vi "Translator.vi"(0 "Input":variant, 11 "error in (no error)":errorcluster) -> (4 "Output":variant, 15 "error out":errorcluster)   [LabVIEW 2014, in "Arduino Extra Functions.lvlib"]
doc: "An example of how to create the Translator to convert the LabVIEW VIs to Arduino C code."
uses:
  <vilib>/Aledyne-TSXperts/Arduino Compatible Compiler for LabVIEW/addons/Arduino Extra Functions/Arduino Extra Functions.lvlib
panel:
  out "Outputs":string[](array[string])
  out "Inputs":string[](array[string])
  out "Output Datatypes":string[](array[string])
  out "Input Datatypes":string[](array[string])
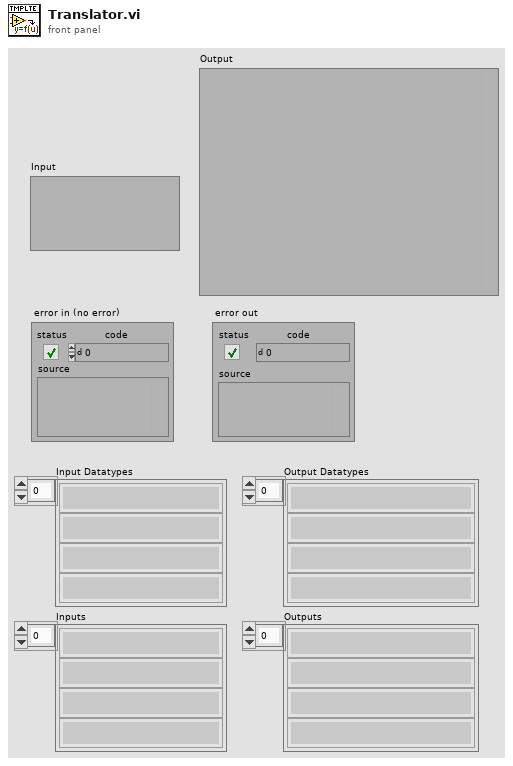
[diagram p1: front panel]
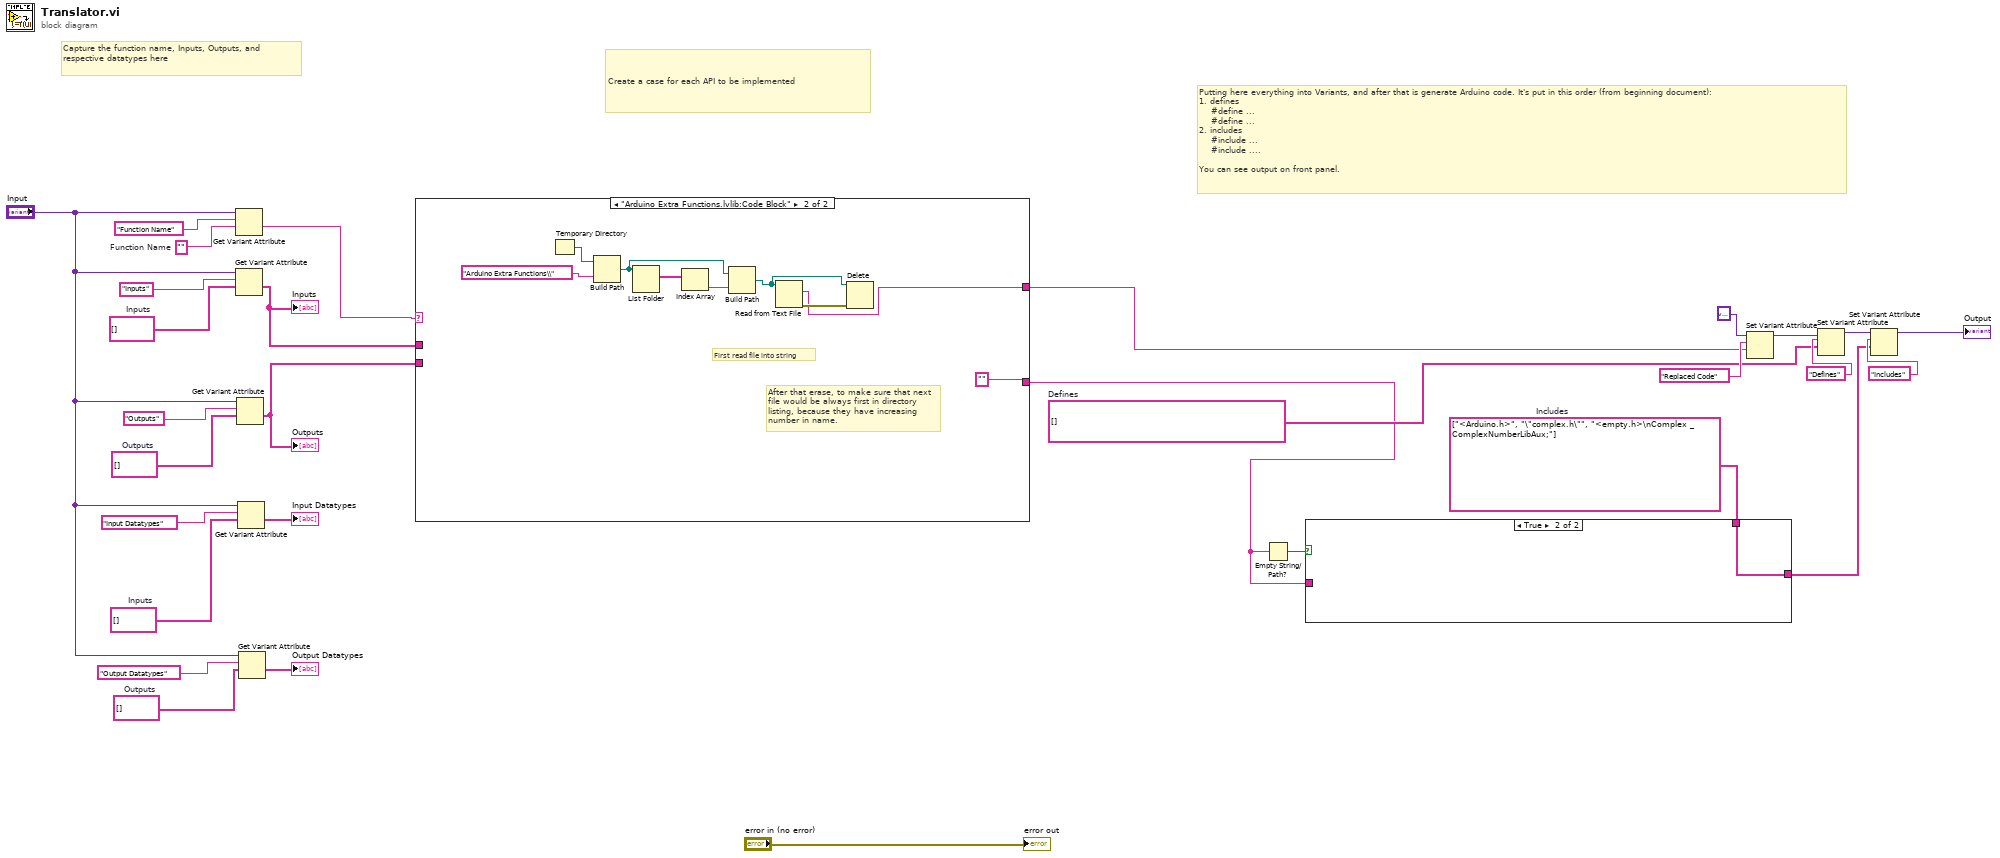
[diagram p0: block diagram]
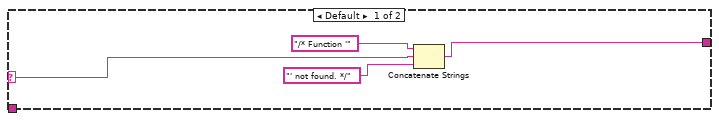
[diagram p2: hidden frame]
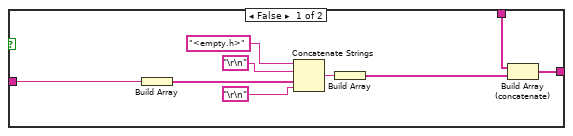
[diagram p3: hidden frame]
diagram:
  w8 = string[] []  # Defines
  w19 = string[] []  # Outputs
  w20 = string[] []  # Inputs
  w6 = string[] ["<Arduino.h>", "\"complex.h\"", "<empty.h>\nComplex _ComplexNumberLibAux;"]  # Includes
  w26 = string[] []  # Outputs
  w27 = string[] []  # Inputs
  w28 = ""  # Function Name
  # "Capture the function name, Inputs, Outputs, and respective datatypes here"
  # "Putting here everything into Variants, and after that is generate Arduino code. It's put in this order (from beginning document):\n1. defines\n    #define ...\n    #define ...\n2. includes\n    #include ...\n    #include ....\n\nYou can see output on front panel."
  # "Create a case for each API to be implemented"
  n1 = Get Variant Attribute(Variant="Input", name="Function Name", default value (empty Variant)=w28) -> (value=w5:string)  [unwired: 1 in, 3 out]
  n2 = Get Variant Attribute(Variant="Input", name="Inputs", default value (empty Variant)=w27) -> (value=w4:string[])  [unwired: 1 in, 3 out]
  "Inputs" <- w4
  n3 = Get Variant Attribute(Variant="Input", name="Outputs", default value (empty Variant)=w26) -> (value=w3:string[])  [unwired: 1 in, 3 out]
  "Outputs" <- w3
  n4 = Get Variant Attribute(Variant="Input", name="Input Datatypes", default value (empty Variant)=w20) -> (value=→"Input Datatypes":string[])  [unwired: 1 in, 3 out]
  n5 = Get Variant Attribute(Variant="Input", name="Output Datatypes", default value (empty Variant)=w19) -> (value=→"Output Datatypes":string[])  [unwired: 1 in, 3 out]
  n6 = case shown="\"Arduino Extra Functions.lvlib:Code Block\"" w5 {
    selector: w5 -> [w34 _]
    tunnel: w4 -> [_ _]
    tunnel: w3 -> [_ _]
    tunnel: [_ ""] -> w2
    tunnel: [w31 w35] -> w1
    frame Default {
      n7 = Concatenate Strings("/* Function '", w34, "' not found. */") -> (w31:string)
    }
    frame "Arduino Extra Functions.lvlib:Code Block" {
      # "After that erase, to make sure that next\nfile would be always first in directory\nlisting, because they have increasing\nnumber in name."
      # "First read file into string"
      n8 = Temporary Directory() -> (w42:path)
      n9 = Build Path(base path=w42, name or relative path="Arduino Extra Functions\\" ("string")) -> (appended path=w38:path)
      n10 = List Folder(path=w38) -> (filenames=w40:string[])  [unwired: 3 in, 3 out]
      n11 = Index Array(array=w40) -> (element=w39:string)  [unwired: 1 in]
      n12 = Build Path(base path=w38, name or relative path=w39) -> (appended path=w36:path)
      n13 = Read from Text File(file (use dialog)=w36) -> (text=w35:string, error out=w37:errorcluster)  [unwired: 3 in, 2 out]
      n14 = Delete(path (use dialog)=w36, error in=w37) -> ()  [unwired: 3 in, 3 out]
    }
  }
  n15 = Empty String/Path?(string/path=w2) -> (empty?=w9:bool)
  n16 = case shown="True" w9 {
    tunnel: w2 -> [w52 _]
    tunnel: [w45 w53] -> w7
    tunnel: w6 -> [w44 w53]
    frame False {
      n17 = Build Array(w52) -> (w46:string[])
      n18 = Concatenate Strings("<empty.h>" ("string"), "\r\n", w46, "\r\n") -> (w47:string)
      n19 = Build Array(w47) -> (w51:string[])
      n20 = Build Array (concatenate)(w44, w51) -> (w45:string[])
    }
    frame True {
    }
  }
  n21 = Set Variant Attribute(Variant=variant ("variant"), name="Replaced Code", value=w1) -> (Variant out=w13:variant)  [unwired: 1 in, 2 out]
  n22 = Set Variant Attribute(Variant=w13, name="Defines", value=w8) -> (Variant out=w12:variant)  [unwired: 1 in, 2 out]
  n23 = Set Variant Attribute(Variant=w12, name="Includes", value=w7) -> (Variant out=→"Output":variant)  [unwired: 1 in, 2 out]
  "error out" <- "error in (no error)"
